vi "Dispose.vi"(8 "error in (no error)":errorcluster, 11 "Server Fixture in":refnum<class "Server Fixture.lvclass">) -> (0 "error out":errorcluster, 4 "Server Standard Error":string, 6 "Server Standard Output":string)   [LabVIEW 2013, in "libssh2_integration_tests.lvlib" / "Server Fixture.lvclass"]
uses:
  Server Fixture.lvclass
  Server Fixture.lvclass/Server Fixture.ctl
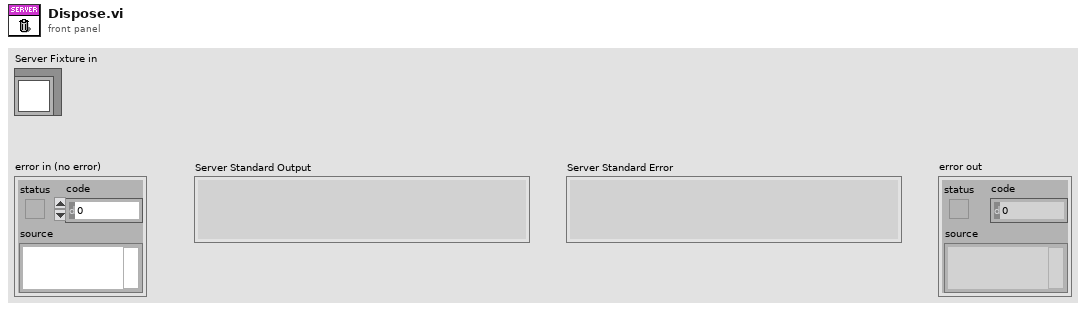
[diagram p1: front panel]
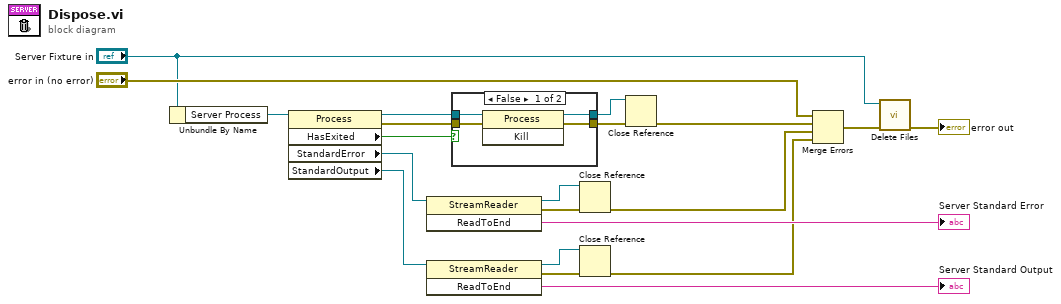
[diagram p0: block diagram]
diagram:
  n1 = Unbundle By Name("Server Fixture in") -> ("Server Process"=w17:refnum<k24>)
  n2 = property class="Process"(reference=w17) -> (reference out=w16:refnum<k24>, error out=w12:errorcluster, "HasExited"=w1:bool, "StandardError"=w15:refnum<k24>, "StandardOutput"=w6:refnum<k24>)  [unwired: 1 in]
  n3 = invoke class="StreamReader" method="ReadToEnd"(reference=w15) -> (reference out=w13:refnum<k24>, error out=w11:errorcluster, "ReadToEnd"=→"Server Standard Error":string)  [unwired: 2 in]
  n4 = invoke class="StreamReader" method="ReadToEnd"(reference=w6) -> (reference out=w7:refnum<k24>, error out=w9:errorcluster, "ReadToEnd"=→"Server Standard Output":string)  [unwired: 2 in]
  n5 = case shown="False" w1 {
    tunnel: [w25 w26] -> w20
    tunnel: [w24 w27] -> w18
    tunnel: w16 -> [w23 w27]
    tunnel: w12 -> [w22 w26]
    frame False {
      n6 = invoke class="Process" method="Kill"(reference=w23, error in=w22) -> (reference out=w24:refnum<k24>, error out=w25:errorcluster)  [unwired: 1 in, 1 out]
    }
    frame True {
    }
  }
  n7 = Close Reference(reference=w13, error in (no error)=w11) -> (error out=w10:errorcluster)
  n8 = Close Reference(reference=w7, error in (no error)=w9) -> (error out=w5:errorcluster)
  n9 = Close Reference(reference=w18, error in (no error)=w20) -> (error out=w19:errorcluster)
  n10 = Merge Errors("error in (no error)", w19, w10, w5) -> (w21:errorcluster)
  n11 = call "Delete Files.vi"("error in (no error)"=w21, "Server Fixture in"="Server Fixture in") -> ("error out"=→"error out":errorcluster)  [unwired: 8 in, 1 out]
